vi "Remove FullyCustom Profile RTM.vi"(8 "error in (no error)":errorcluster, 11 "Node Ptr":u64 format="%.0x") -> (0 "error out":errorcluster)   [LabVIEW 2011, in "Engine Sim System Explorer.lvlib"]
uses:
  Engine Sim System Explorer.lvlib
  <vilib>/NI Veristand/Custom Device API/Custom Device API.lvlib
  <vilib>/NI Veristand/Custom Device Tools/Custom Device Utility Library/Custom Device Utility Library.lvlib
panel:
  in  "Tag":string
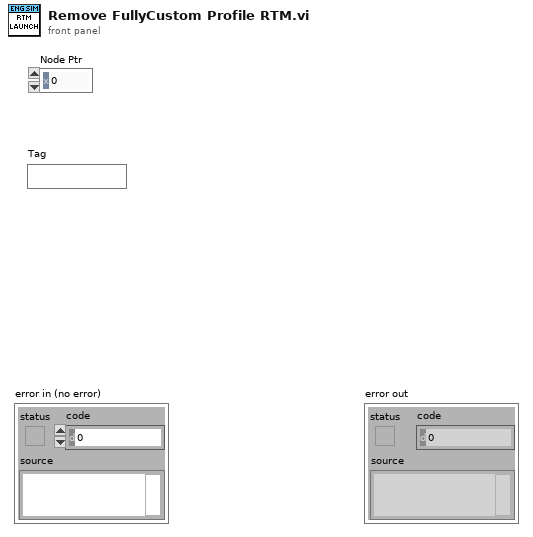
[diagram p1: front panel]
types:
  T1 = typedef "Custom Device API.lvlib/Custom Device Item Ref.ctl" = u64
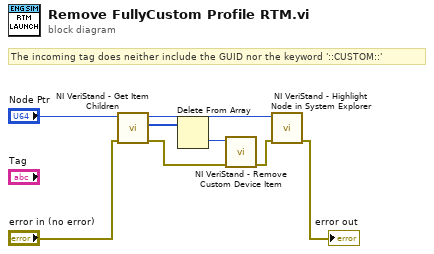
[diagram p0: block diagram]
diagram:
  # "The incoming tag does neither include the GUID nor the keyword '::CUSTOM::'"
  n1 = call <vilib>:"NI VeriStand - Get Item Children.vi"("error in (no error)"="error in (no error)", "Item Ref in"="Node Ptr") -> ("error out"=w4:errorcluster, "Child Refs"=w6:T1[], "Item Ref out"=w3:T1)  [unwired: 6 in, 1 out]
  n2 = Delete From Array(array=w6) -> (deleted portion=w5:T1)  [unwired: 2 in, 1 out]
  n3 = call <vilib>:"NI VeriStand - Remove Custom Device Item.vi"("error in (no error)"=w4, "Item Ref in"=w5) -> ("error out"=w2:errorcluster)  [unwired: 8 in, 1 out]
  n4 = call <vilib>:"NI VeriStand - Highlight Node in System Explorer.vi"("error in (no error)"=w2, "Item Ref in"=w3) -> ("error out"=→"error out":errorcluster)  [unwired: 8 in, 1 out]
